vi "Autonomous Independent.vi"   [LabVIEW 2013]
doc: "This VI is called when autonomous begins, and will automatically be terminated when autonomous ends. You can carry out timed or sensor driven robot movement independently without needing to return to the caller."
uses:
  Robot Global Data.vi
  <vilib>/Rock Robotics/WPI/RobotDrive/WPI_RobotDriveGetSetRefNum.vi
  <vilib>/Rock Robotics/WPI/Joystick/WPI_JoystickGetSetRefNum.vi
  <vilib>/Rock Robotics/WPI/RobotDrive/WPI_RobotDriveMecanumDrive_Cartesian.vi
panel:
  # "Be sure to right-click and choose Data Operations>>Make Current Value default if you want to save the array values with the VI"
types:
  T1 = typedef "WPI_JoystickDevRef.ctl" = cluster{"Device":T2}
  T2 = typedef "WPI_JoystickDeviceEnum.ctl" = enum16{"USB 1", "USB 2", "USB 3", "USB 4", "Kinect 1", "Kinect 2"}
  T3 = cluster{"axis 1 (x)":dbl, "axis 2 (y)":dbl, "axis 3 (throttle)":dbl, "axis 4":dbl, "axis 5":dbl, "axis 6":dbl}
  T4 = typedef "WPI_RobotDriveDevRef.ctl" = cluster{"DevStatus":errorcluster, "Motors[]":T5[], "Square Inputs":bool, "Max Output":dbl, "Isochronous":bool}
  T5 = typedef "WPI_MotorControlDeviceRef.ctl" = cluster{"DeviceStatus":errorcluster, "Type":enum16{"PWM", "CAN"}, "PWM":cluster{"Digital Module":T6, "PWM Channel":T7, "DeadBand":T8}, "CAN":cluster{"Device Number":u8, "Control Mode":T9, "Semaphore":T10, "Max Vout":dbl}, "Invert":bool, "TransformRef":T11, "InvTransformRef":T11}
  T6 = typedef "FPGA_TypedefDigitalModule.ctl" = enum16{"Digital Module 1", "Digital Module 2"}
  T7 = typedef "FPGA_DIOPWMChannel.ctl" = enum8{"PWM 1", "PWM 2", "PWM 3", "PWM 4", "PWM 5", "PWM 6", "PWM 7", "PWM 8", "PWM 9", "PWM 10", "Invalid"}
  T8 = typedef "WPI_PWMDeadband.ctl" = cluster{"Name":string, "maxPositivePwm":i32, "minPositivePwm":i32, "centerPwm":i32, "maxNegativePwm":i32, "minNegativePwm":i32, "angularRange":u16}
  T9 = typedef "WPI_CANJaguar_ControlMode.ctl" = enum8{"Percent VBus", "Current", "Speed", "Position", "Voltage"}
  T10 = typedef "Semaphore RefNum" = refnum<k1>
  T11 = typedef "WPI_PWMTransform_ConPane.ctl" = refnum<vi>
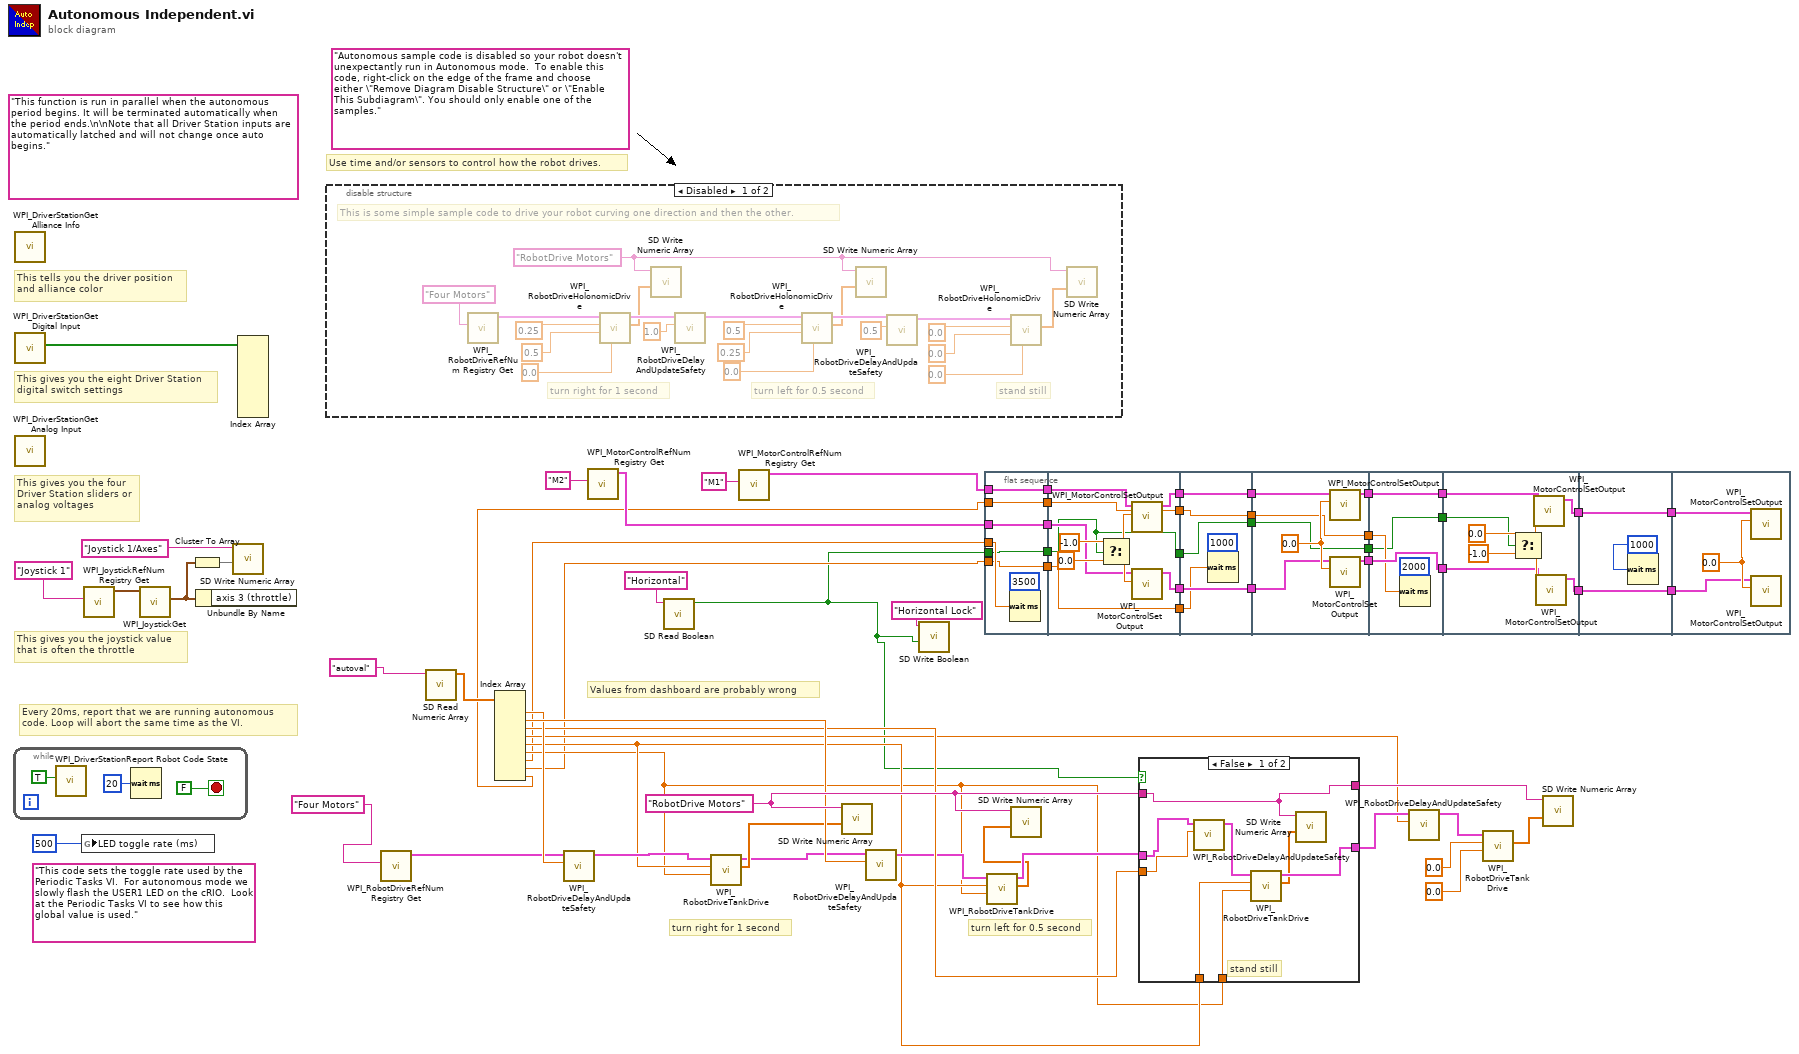
[diagram p0: block diagram]
diagram:
  w33 = "RobotDrive Motors" ("Name")
  (unwired) "This code sets the toggle rate used by the Periodic Tasks VI.  For autonomous mode we slowly flash the USER1 LED on the cRIO.  Look at the Periodic Tasks VI to see how this global value is used."
  (unwired) "Autonomous sample code is disabled so your robot doesn't unexpectantly run in Autonomous mode.  To enable this code, right-click on the edge of the frame and choose either \"Remove Diagram Disable Structure\" or \"Enable This Subdiagram\". You should only enable one of the samples."
  (unwired) "This function is run in parallel when the autonomous period begins. It will be terminated automatically when the period ends.\n\nNote that all Driver Station inputs are automatically latched and will not change once auto begins."
  # "Values from dashboard are probably wrong"
  # "turn left for 0.5 second"
  # "turn right for 1 second"
  # "Every 20ms, report that we are running autonomous\ncode. Loop will abort the same time as the VI."
  # "This gives you the joystick value\nthat is often the throttle"
  # "Use time and/or sensors to control how the robot drives."
  # "This tells you the driver position\nand alliance color"
  # "This gives you the eight Driver Station\ndigital switch settings"
  # "This gives you the four\nDriver Station sliders or\nanalog voltages"
  n1 = while {
    stop <- FALSE stop-if-true
    n2 = call <vilib>:"WPI_DriverStationReport Robot Code State.vi"("Autonomous"=TRUE) -> ()  [unwired: 10 in, 1 out]
    n3 = Wait (ms)(milliseconds to wait=u32 20) -> ()  [unwired: 1 out]
  }
  n4 = call <vilib>:"WPI_DriverStationGet Alliance Info.vi"() -> ()  [unwired: 12 out]
  n5 = call <vilib>:"WPI_DriverStationGet Digital Input.vi"() -> ("Driver Station Digital Input (1-8)"=w65:bool[])  [unwired: 11 out]
  n6 = call <vilib>:"WPI_DriverStationGet Analog Input.vi"() -> ()  [unwired: 12 out]
  n7 = global write "Robot Global Data.vi" "LED toggle rate (ms)"(u32 500 ("LED ms toggle rate")) -> ()
  n8 = call <vilib>:"WPI_JoystickRefNum Registry Get.vi"("refnum name"="Joystick 1") -> ("JoystickDevRef"=w63:T1)  [unwired: 1 in, 9 out]
  n9 = call <vilib>:"WPI_JoystickGet.vi"("JoystickDevRef"=w63) -> ("Axes"=w60:T3)  [unwired: 1 in, 5 out]
  n10 = Cluster To Array(cluster=w60) -> (array=w61:dbl[])
  n11 = Unbundle By Name(w60) -> ()  [unwired: 1 out]
  n12 = call <vilib>:"SD Write Numeric Array.vi"("Numeric Array"=w61, "Name"="Joystick 1/Axes") -> ()  [unwired: 8 in, 2 out]
  n13 = Index Array(array=w65) -> ()  [unwired: 8 in, 8 out]
  n14 = disable-structure shown="Disabled" {
    frame Disabled {
      w72 = "RobotDrive Motors" ("Name")
      # "This is some simple sample code to drive your robot curving one direction and then the other."
      # "stand still"
      # "turn left for 0.5 second"
      # "turn right for 1 second"
      n15 = call <vilib>:"WPI_RobotDriveRefNum Registry Get.vi"("refnum name"="Four Motors") -> ("RobotDriveDevRef"=w76:T4)  [unwired: 1 in, 9 out]
      n16 = call-poly <vilib>:"WPI_RobotDriveHolonomicDrive.vi"("Rotation"=0.0, "Y"=0.5 ("X axis value"), "X"=0.25 ("X axis value"), "RobotDriveDevRef"=w76) -> ("Motor Values"=w75:dbl[], "RobotDriveDevRef"=w83:T4)  [unwired: 5 in, 1 out]
      n17 = call <vilib>:"SD Write Numeric Array.vi"("Numeric Array"=w75, "Name"=w72) -> ()  [unwired: 8 in, 2 out]
      n18 = call <vilib>:"WPI_RobotDriveDelayAndUpdateSafety.vi"("Delay (s)"=1.0, "RobotDriveDevRef"=w83) -> ("RobotDriveDevRef 2"=w82:T4)  [unwired: 8 in, 1 out]
      n19 = call-poly <vilib>:"WPI_RobotDriveHolonomicDrive.vi"("Rotation"=0.0, "Y"=0.25 ("X axis value"), "X"=0.5 ("X axis value"), "RobotDriveDevRef"=w82) -> ("Motor Values"=w74:dbl[], "RobotDriveDevRef"=w81:T4)  [unwired: 5 in, 1 out]
      n20 = call <vilib>:"SD Write Numeric Array.vi"("Numeric Array"=w74, "Name"=w72) -> ()  [unwired: 8 in, 2 out]
      n21 = call <vilib>:"WPI_RobotDriveDelayAndUpdateSafety.vi"("Delay (s)"=0.5, "RobotDriveDevRef"=w81) -> ("RobotDriveDevRef 2"=w80:T4)  [unwired: 8 in, 1 out]
      n22 = call-poly <vilib>:"WPI_RobotDriveHolonomicDrive.vi"("Rotation"=0.0 ("X axis value"), "Y"=0.0 ("X axis value"), "X"=0.0 ("X axis value"), "RobotDriveDevRef"=w80) -> ("Motor Values"=w73:dbl[])  [unwired: 5 in, 2 out]
      n23 = call <vilib>:"SD Write Numeric Array.vi"("Numeric Array"=w73, "Name"=w72) -> ()  [unwired: 8 in, 2 out]
    }
    frame Enabled {
    }
  }
  n24 = call <vilib>:"WPI_RobotDriveRefNum Registry Get.vi"("refnum name"="Four Motors") -> ("RobotDriveDevRef"=w17:T4)  [unwired: 1 in, 9 out]
  n25 = call <vilib>:"SD Read Numeric Array.vi"("Name"="autoval") -> ("Numeric Array"=w30:dbl[])  [unwired: 8 in, 2 out]
  n26 = Index Array(array=w30) -> (element #1=w25:dbl, element #2=w29:dbl, element #3=w24:dbl, element #4=w20:dbl, element #5=w15:dbl, element #6=w14:dbl, element #7=w5:dbl, element #8=w4:dbl, element #9=w3:dbl)  [unwired: 9 in]
  n27 = call <vilib>:"WPI_RobotDriveDelayAndUpdateSafety.vi"("Delay (s)"=w25, "RobotDriveDevRef"=w17) -> ("RobotDriveDevRef 2"=w27:T4)  [unwired: 8 in, 1 out]
  n28 = call <vilib>:"WPI_MotorControlRefNum Registry Get.vi"("refnum name"="M2") -> ("MotorControlDevRef"=w6:T5)  [unwired: 9 in, 1 out]
  n29 = call <vilib>:"SD Read Boolean.vi"("Name"="Horizontal") -> ("Boolean"=w2:bool)  [unwired: 8 in, 2 out]
  n30 = call <vilib>:"WPI_RobotDriveTankDrive.vi"("Right axis value"=w14, "Left axis value"=w15, "RobotDriveDevRef"=w27) -> ("Motor Values"=w28:dbl[], "RobotDriveDevRef"=w26:T4)  [unwired: 6 in, 1 out]
  n31 = call <vilib>:"WPI_MotorControlRefNum Registry Get.vi"("refnum name"="M1") -> ("MotorControlDevRef"=w7:T5)  [unwired: 9 in, 1 out]
  n32 = call <vilib>:"SD Write Numeric Array.vi"("Numeric Array"=w28, "Name"=w33) -> ()  [unwired: 8 in, 2 out]
  n33 = call <vilib>:"WPI_RobotDriveDelayAndUpdateSafety.vi"("Delay (s)"=w29, "RobotDriveDevRef"=w26) -> ("RobotDriveDevRef 2"=w23:T4)  [unwired: 8 in, 1 out]
  n34 = call <vilib>:"SD Write Boolean.vi"("Boolean"=w2, "Name"="Horizontal Lock") -> ()  [unwired: 8 in, 2 out]
  n35 = flat-sequence {
    tunnel: w5 -> [w95]
    tunnel: w4 -> [w94]
    tunnel: [w94] -> w58
    tunnel: w3 -> [w93]
    tunnel: [w93] -> w57
    tunnel: w7 -> [w92]
    tunnel: [w92] -> w56
    tunnel: w6 -> [w91]
    tunnel: [w91] -> w55
    tunnel: w2 -> [w90]
    tunnel: [w90] -> w54
    tunnel: [w102] -> w53
    tunnel: [w101] -> w52
    tunnel: w58 -> [w100]
    tunnel: [w100] -> w51
    tunnel: w57 -> [w99]
    tunnel: [w99] -> w50
    tunnel: w56 -> [w98]
    tunnel: w55 -> [w97]
    tunnel: w54 -> [w96]
    tunnel: [w96] -> w49
    tunnel: [w110] -> w48
    tunnel: w53 -> [w110]
    tunnel: [w109] -> w47
    tunnel: w52 -> [w109]
    tunnel: w51 -> [w108]
    tunnel: w50 -> [w107]
    tunnel: [w107] -> w46
    tunnel: w49 -> [w106]
    tunnel: [w106] -> w45
    tunnel: w48 -> [w116]
    tunnel: w47 -> [w115]
    tunnel: [w114] -> w44
    tunnel: [w113] -> w43
    tunnel: w46 -> [w112]
    tunnel: [w112] -> w42
    tunnel: w45 -> [w111]
    tunnel: [w111] -> w41
    tunnel: [w121] -> w40
    tunnel: w44 -> [w121]
    tunnel: [w120] -> w39
    tunnel: w43 -> [w120]
    tunnel: w42 -> [w119]
    tunnel: [w118] -> w38
    tunnel: w41 -> [w118]
    tunnel: w40 -> [w126]
    tunnel: w39 -> [w125]
    tunnel: [w124] -> w37
    tunnel: [w123] -> w36
    tunnel: w38 -> [w122]
    tunnel: [w131] -> w35
    tunnel: w37 -> [w131]
    tunnel: [w130] -> w34
    tunnel: w36 -> [w130]
    tunnel: w35 -> [w134]
    tunnel: w34 -> [w133]
    frame #0 {
      (unwired) 3500
      n36 = Wait (ms)(milliseconds to wait=w95) -> ()  [unwired: 1 out]
    }
    frame #1 {
      n37 = Select(t=-1.0, s=w96, f=0.0) -> (s? t:f=w105:dbl)
      n38 = call <vilib>:"WPI_MotorControlSetOutput.vi"("Output"=w105, "MotorControlDevRef"=w98) -> ("MotorControlDevRef"=w102:T5)  [unwired: 7 in, 2 out]
      n39 = call <vilib>:"WPI_MotorControlSetOutput.vi"("Output"=w105, "MotorControlDevRef"=w97) -> ("MotorControlDevRef"=w101:T5)  [unwired: 7 in, 2 out]
    }
    frame #2 {
      (unwired) 1000
      n40 = Wait (ms)(milliseconds to wait=w108) -> ()  [unwired: 1 out]
    }
    frame #3 {
      w117 = 0.0
      n41 = call <vilib>:"WPI_MotorControlSetOutput.vi"("Output"=w117, "MotorControlDevRef"=w116) -> ("MotorControlDevRef"=w114:T5)  [unwired: 7 in, 2 out]
      n42 = call <vilib>:"WPI_MotorControlSetOutput.vi"("Output"=w117, "MotorControlDevRef"=w115) -> ("MotorControlDevRef"=w113:T5)  [unwired: 7 in, 2 out]
    }
    frame #4 {
      (unwired) 2000
      n43 = Wait (ms)(milliseconds to wait=w119) -> ()  [unwired: 1 out]
    }
    frame #5 {
      n44 = Select(t=0.0, s=w122, f=-1.0) -> (s? t:f=w129:dbl)
      n45 = call <vilib>:"WPI_MotorControlSetOutput.vi"("Output"=w129, "MotorControlDevRef"=w126) -> ("MotorControlDevRef"=w124:T5)  [unwired: 7 in, 2 out]
      n46 = call <vilib>:"WPI_MotorControlSetOutput.vi"("Output"=w129, "MotorControlDevRef"=w125) -> ("MotorControlDevRef"=w123:T5)  [unwired: 7 in, 2 out]
    }
    frame #6 {
      n47 = Wait (ms)(milliseconds to wait=1000) -> ()  [unwired: 1 out]
    }
    frame #7 {
      w135 = 0.0
      n48 = call <vilib>:"WPI_MotorControlSetOutput.vi"("Output"=w135, "MotorControlDevRef"=w134) -> ()  [unwired: 7 in, 3 out]
      n49 = call <vilib>:"WPI_MotorControlSetOutput.vi"("Output"=w135, "MotorControlDevRef"=w133) -> ()  [unwired: 7 in, 3 out]
    }
  }
  n50 = call <vilib>:"WPI_RobotDriveTankDrive.vi"("Right axis value"=w14, "Left axis value"=w15, "RobotDriveDevRef"=w23) -> ("Motor Values"=w21:dbl[], "RobotDriveDevRef"=w22:T4)  [unwired: 6 in, 1 out]
  n51 = call <vilib>:"SD Write Numeric Array.vi"("Numeric Array"=w21, "Name"=w33) -> ()  [unwired: 8 in, 2 out]
  n52 = case shown="False" w2 {
    tunnel: w33 -> [w142 w145]
    tunnel: w22 -> [w143 w144]
    tunnel: [w139 w144] -> w31
    tunnel: [w142 w145] -> w32
    tunnel: w24 -> [w141 _]
    tunnel: w15 -> [w137 _]
    tunnel: w14 -> [w136 _]
    frame False {
      # "stand still"
      n53 = call <vilib>:"WPI_RobotDriveDelayAndUpdateSafety.vi"("Delay (s)"=w141, "RobotDriveDevRef"=w143) -> ("RobotDriveDevRef 2"=w140:T4)  [unwired: 8 in, 1 out]
      n54 = call <vilib>:"WPI_RobotDriveTankDrive.vi"("Right axis value"=w136, "Left axis value"=w137, "RobotDriveDevRef"=w140) -> ("Motor Values"=w138:dbl[], "RobotDriveDevRef"=w139:T4)  [unwired: 6 in, 1 out]
      n55 = call <vilib>:"SD Write Numeric Array.vi"("Numeric Array"=w138, "Name"=w142) -> ()  [unwired: 8 in, 2 out]
    }
    frame True {
    }
  }
  n56 = call <vilib>:"WPI_RobotDriveDelayAndUpdateSafety.vi"("Delay (s)"=w20, "RobotDriveDevRef"=w31) -> ("RobotDriveDevRef 2"=w19:T4)  [unwired: 8 in, 1 out]
  n57 = call <vilib>:"WPI_RobotDriveTankDrive.vi"("Right axis value"=0.0, "Left axis value"=0.0, "RobotDriveDevRef"=w19) -> ("Motor Values"=w18:dbl[])  [unwired: 6 in, 2 out]
  n58 = call <vilib>:"SD Write Numeric Array.vi"("Numeric Array"=w18, "Name"=w32) -> ()  [unwired: 8 in, 2 out]
